vi "Update.vi"(8 "error in (no error)":errorcluster, 10 "Numeric":dbl, 11 "RealBattery in":refnum<class "RealBattery.lvclass">) -> (0 "error out":errorcluster, 3 "RealBattery out":refnum<class "RealBattery.lvclass">)   [LabVIEW 2011, in "RealBattery.lvclass"]
uses:
  RealBattery.lvclass
  Abstract Battery/AbstractBattery.lvclass
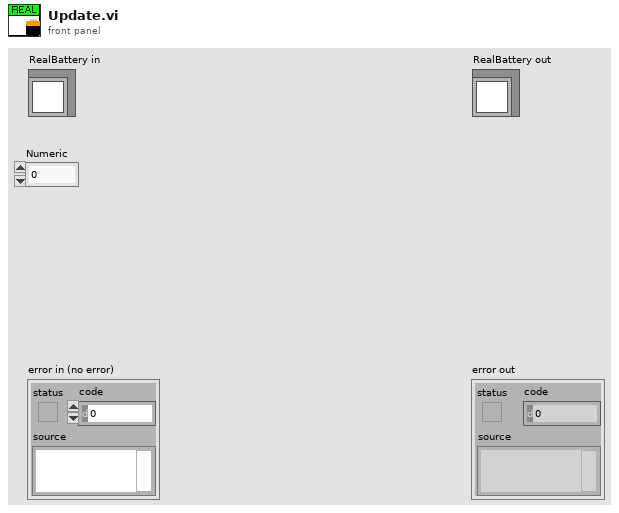
[diagram p1: front panel]
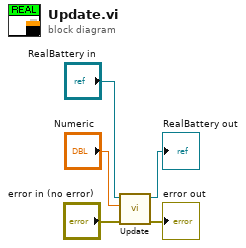
[diagram p0: block diagram]
diagram:
  n1 = call-parent "Update.vi"("error in (no error)"="error in (no error)", "Numeric"="Numeric", "AbstractBattery in"="RealBattery in") -> ("error out"=→"error out":errorcluster, "AbstractBattery out"=→"RealBattery out":refnum<class "RealBattery.lvclass">)  [unwired: 7 in]
